vi "DisplayErrorInEngineDialog.vi"(8 "error in (no error)":errorcluster, 10 "TestStand Engine":refnum<k7>) -> ()   [LabVIEW 2023, in "GUI.lvlib" / "Auto UI.lvlib" / "Auto UI.lvclass"]
uses:
  Auto UI.lvclass
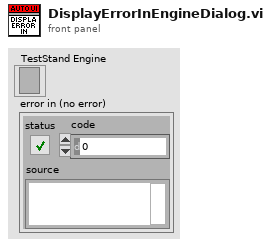
[diagram p1: front panel]
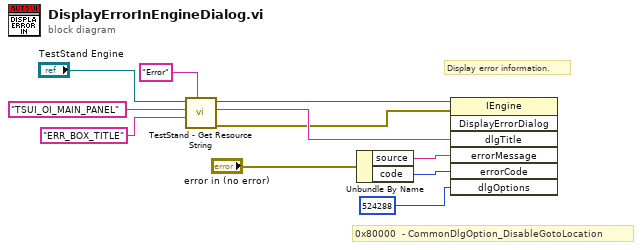
[diagram p0: block diagram]
diagram:
  # "0x80000  - CommonDlgOption_DisableGotoLocation"
  # "Display error information."
  n1 = call <vilib>:"TestStand - Get Resource String.vi"("Default String"="Error", "Symbol"="ERR_BOX_TITLE", "Category"="TSUI_OI_MAIN_PANEL", "Engine Reference In"="TestStand Engine") -> ("error out"=w6:errorcluster, "Resource String"=w8:string, "Engine Reference Out"=w7:refnum<k7>)  [unwired: 1 in, 4 out]
  n2 = Unbundle By Name("error in (no error)") -> ("source"=w3:string, "code"=w2:i32)
  n3 = invoke class="IEngine" method="DisplayErrorDialog"(reference=w7, error in=w6, "dlgTitle"=w8, "errorMessage"=w3, "errorCode"=w2, "dlgOptions"=524288) -> ()  [unwired: 1 in, 7 out]
